vi "Generate TimerUserEvent.vi"(10 "TimePeroid(ms)":i32, 11 "TimerEngine in":refnum<class "TimerEngine.lvclass">) -> (2 "UserEvent":T1, 3 "TimerEngine out":refnum<class "TimerEngine.lvclass">)   [LabVIEW 2017, in "TimerEngine.lvlib" / "TimerEngine.lvclass"]
uses:
  TimerEngine.lvclass
  _Typedef/Timer-UserEvent.ctl
  TimerEngine.lvclass/TimerEngine.ctl
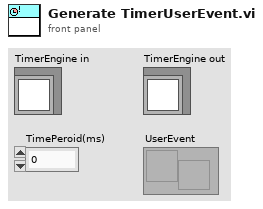
[diagram p1: front panel]
types:
  T1 = typedef "TimerEngine.lvlib/TimerEngine.lvclass/Timer-UserEvent.ctl" = refnum<user-event>
  T2 = typedef "TimerEngine.lvlib/TimerEngine.lvclass/Timer-Userevent.ctl" = refnum<user-event>
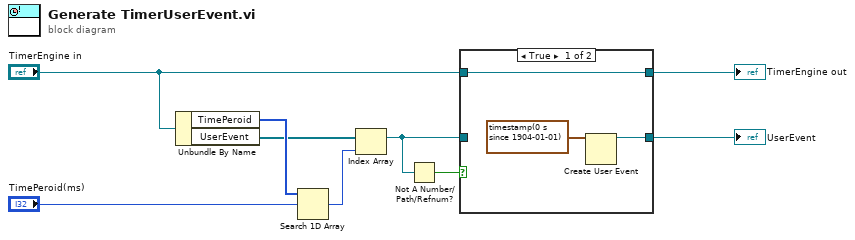
[diagram p0: block diagram]
diagram:
  n1 = Unbundle By Name("TimerEngine in") -> ("TimePeroid"=w3:i32[], "UserEvent"=w1:T2[])
  n2 = Search 1D Array(1D array=w3, element="TimePeroid(ms)") -> (index of element=w4:i32)  [unwired: 1 in]
  n3 = Index Array(array=w1, index=w4) -> (element=w5:T2)
  n4 = Not A Number/Path/Refnum?(number/path/refnum=w5) -> (NaN/Path/Refnum?=w6:bool)
  n5 = case shown="True" w6 {
    tunnel: w5 -> [_ w13]
    tunnel: "TimerEngine in" -> [w11 w14]
    tunnel: [w10 w13] -> w8
    tunnel: [w11 w14] -> w7
    frame True {
      n6 = Create User Event(user event datatype=timestamp(0 s since 1904-01-01) ("Time Stamp")) -> (user event=w10:refnum<user-event>)  [unwired: 1 in, 1 out]
    }
    frame False {
    }
  }
  "UserEvent" <- w8
  "TimerEngine out" <- w7
